vi "Error(s) To Strings.vi"(8 "error in (no error)":errorcluster) -> (2 "Error Strings":string[](array[string]))   [LabVIEW 2020, in "Multiple Errors.lvclass"]
uses:
  Multiple Errors.lvclass
  <vilib>/Utility/error.llb/DialogTypeEnum.ctl
  <vilib>/MultiError/TokenizeJSON/Multi Error Cluster.lvlib
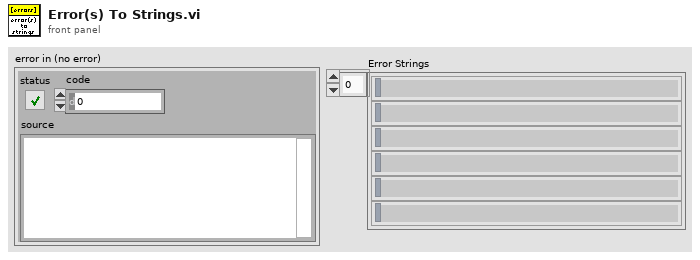
[diagram p1: front panel]
types:
  T1 = typedef "DialogTypeEnum.ctl" = enum16{"no dialog", "OK message", "continue or stop message", "auto error handling dialog", "OK message + warnings", "continue/stop + warnings"}
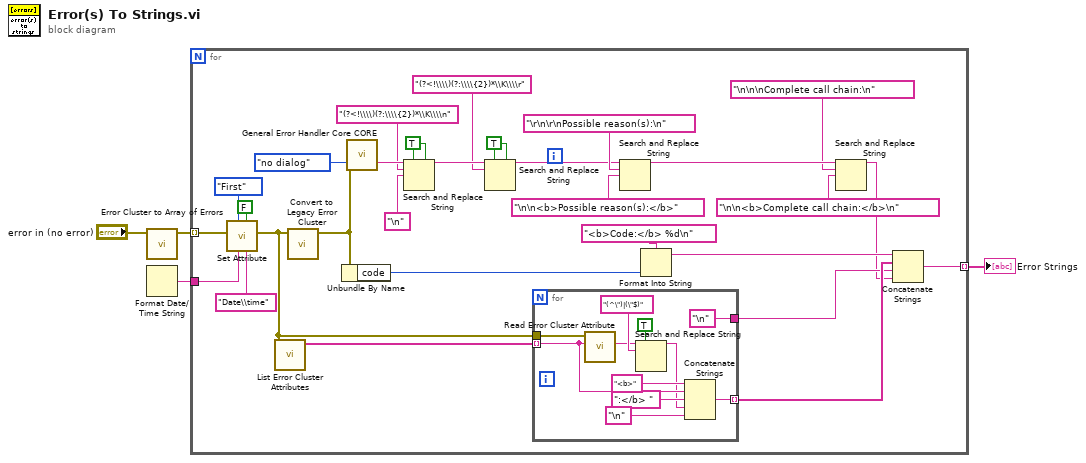
[diagram p0: block diagram]
diagram:
  n1 = call <vilib>:"Error Cluster to Array of Errors.vi"("error"="error in (no error)") -> ("array of errors"=w2:errorcluster[])  [unwired: 10 in]
  n2 = Format Date/Time String() -> (date/time string=w3:string)  [unwired: 3 in]
  n3 = for {
    tunnel: w2 -> [w25] mode=indexing
    tunnel: [w20] -> w4 mode=indexing
    tunnel: w3 -> [w23]
    w14 = TRUE ("replace all? (F)")
    w13 = TRUE ("replace all? (F)")
    n4 = call "Set Attribute.vi"("Attribute [\"Info\"]"="Date\\time" ("Attribute [\"Info\"]"), "Overwrite? [T]"=FALSE, "Text"=w23, "Error [Last]"=enum16{"First", "Last", "All"}."First", "error in (no error)"=w25) -> ("error out"=w24:errorcluster)  [unwired: 6 in]
    n5 = call <vilib>:"List Error Cluster Attributes.vi"("error"=w24) -> ("attribute names"=w30:string[])  [unwired: 10 in]
    n6 = call <vilib>:"Convert to Legacy Error Cluster.vi"("error in"=w24) -> ("error out"=w31:errorcluster)  [unwired: 10 in]
    n7 = Unbundle By Name(w31) -> ("code"=w28:i32)
    n8 = call <vilib>:"General Error Handler Core CORE.vi"("type of dialog (OK msg:1)"=DialogTypeEnum."no dialog", "error in (no error)"=w31) -> ("message"=w19:string)  [unwired: 12 in, 5 out]
    n9 = Search and Replace String(replace all?=w13, multiline?=w13, input string=w19, search string="(?<!\\\\)(?:\\\\{2})*\\K\\\\n", replace string="\n") -> (result string=w16:string)  [unwired: 3 in, 3 out]
    n10 = Search and Replace String(replace all?=w14, multiline?=w14, input string=w16, search string="(?<!\\\\)(?:\\\\{2})*\\K\\\\r") -> (result string=w15:string)  [unwired: 4 in, 3 out]
    n11 = for {
      tunnel: w30 -> [w41] mode=indexing
      tunnel: w24 -> [w44]
      tunnel: [w36] -> w29 mode=indexing
      tunnel: ["\n"] -> w11
      n12 = call <vilib>:"Read Error Cluster Attribute.vi"("attribute name"=w41, "error"=w44) -> ("value string"=w38:string)  [unwired: 7 in, 2 out]
      n13 = Search and Replace String(replace all?=TRUE ("replace all? (F)"), input string=w38, search string="(^\")|(\"$)") -> (result string=w37:string)  [unwired: 5 in, 3 out]
      n14 = Concatenate Strings("<b>", w41, ":</b> ", w37, "\n") -> (w36:string)
    }
    n15 = Search and Replace String(input string=w15, search string="\r\n\r\nPossible reason(s):\n", replace string="\n\n<b>Possible reason(s):</b>") -> (result string=w9:string)  [unwired: 5 in, 3 out]
    n16 = Format Into String(format string="<b>Code:</b> %d\n", w28) -> (resulting string=w26:string)  [unwired: 2 in, 1 out]
    n17 = Search and Replace String(input string=w9, search string="\n\n\nComplete call chain:\n", replace string="\n\n<b>Complete call chain:</b>\n") -> (result string=w8:string)  [unwired: 5 in, 3 out]
    n18 = Concatenate Strings(w26, w29, w11, w8) -> (w20:string)
  }
  "Error Strings" <- w4
